vi "FTW-JSON-ObjectManip-AddPair-Integer.vi"(0 "Input JSON Object":string, 5 "Key":string, 7 "Value":i64, 11 "error in":errorcluster) -> (4 "Output JSON Object":string, 15 "error out":errorcluster)   [LabVIEW 2013]
uses:
  FTW-JSON.lvclass
panel:
  # "Inputs"
  # "Outputs"
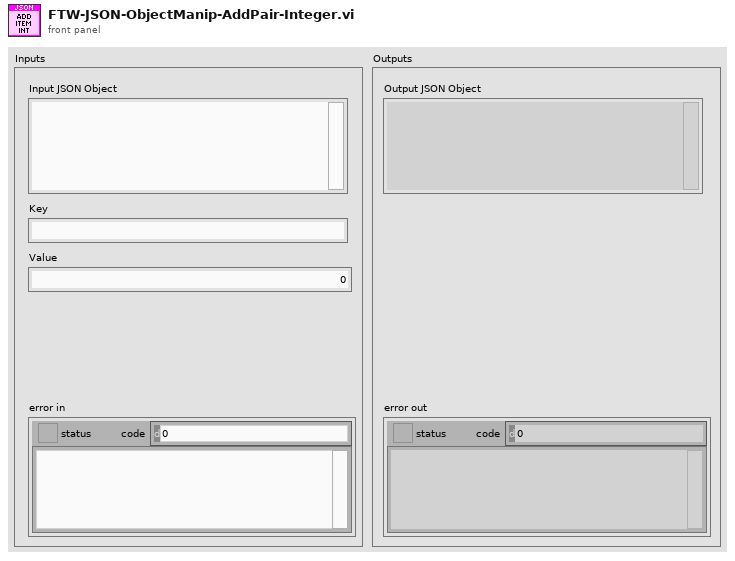
[diagram p1: front panel]
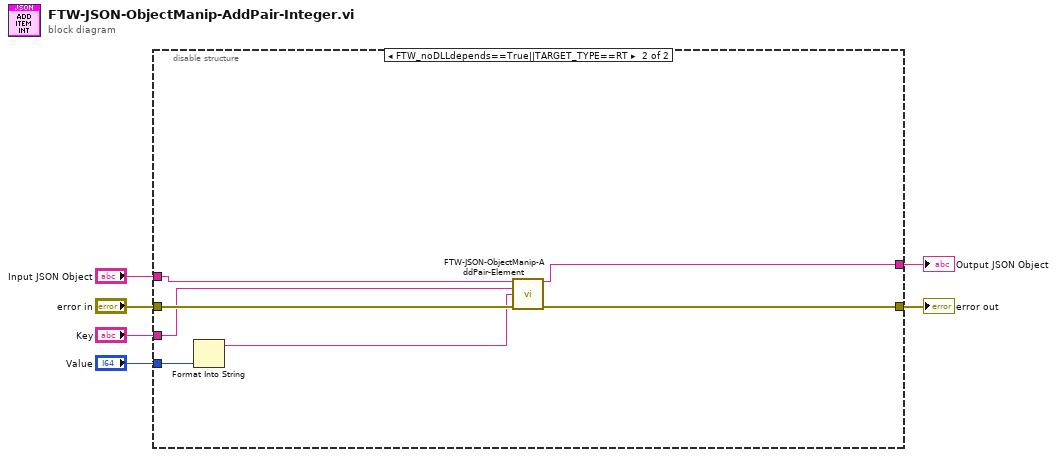
[diagram p0: block diagram]
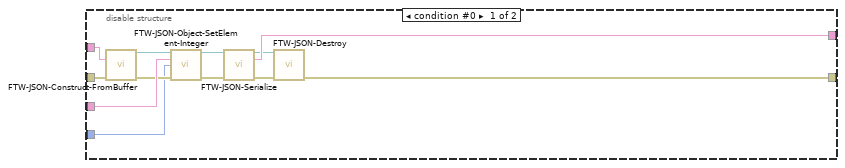
[diagram p2: hidden frame]
diagram:
  n1 = disable-structure shown="FTW_noDLLdepends==True||TARGET_TYPE==RT" {
    disable-tunnel: "Key" -> [w18 w21]
    disable-tunnel: "Value" -> [w7 w20]
    disable-tunnel: "Input JSON Object" -> [w17 w23]
    disable-tunnel: "error in" -> [w16 w25]
    disable-tunnel: [w15 w24] -> w2
    disable-tunnel: [w14 w22] -> w1
    frame condition #0 {
      n2 = call "FTW-JSON-Construct-FromBuffer.vi"("JSON String (UTF-8)"=w17, "error in"=w16) -> ("JSON Object"=w11:refnum<class "FTW-JSON.lvclass">, "error out"=w9:errorcluster)  [unwired: 12 in]
      n3 = call "FTW-JSON-Object-SetElement-Integer.vi"("JSON Object"=w11, "Key"=w18, "Value"=w7, "error in"=w9) -> ("JSON Object out"=w10:refnum<class "FTW-JSON.lvclass">, "error out"=w8:errorcluster)  [unwired: 10 in]
      n4 = call "FTW-JSON-Serialize.vi"("JSON Object"=w10, "error in"=w8) -> ("JSON Object out"=w13:refnum<class "FTW-JSON.lvclass">, "JSON String (UTF-8)"=w14:string, "error out"=w12:errorcluster)  [unwired: 11 in]
      n5 = call "FTW-JSON-Destroy.vi"("JSON Object"=w13, "error in"=w12) -> ("error out"=w15:errorcluster)  [unwired: 13 in]
    }
    frame condition #1 (active) {
      n6 = Format Into String(w20) -> (resulting string=w19:string)  [unwired: 3 in, 1 out]
      n7 = call "FTW-JSON-ObjectManip-AddPair-Element.vi"("Input JSON Object"=w23, "Key"=w21, "Element String"=w19, "error in"=w25) -> ("Output JSON Object"=w22:string, "error out"=w24:errorcluster)  [unwired: 10 in]
    }
  }
  "error out" <- w2
  "Output JSON Object" <- w1
